vi "TCP.IP Server for Ripple Detection - Experiment 2.vi"() -> ()   [LabVIEW 2021]
doc: "Demonstrates how to set up a basic TCP connection, send data to the specified port once a connection has been established, and terminate the connection once the data has been sent. This VI is designed to stop if the TCP connection is terminated. The data sent in this example is an array of random numbers."
panel:
  in  "Number of row to read \nat a time":i32=10000
  in  "File Path":path
  out "Iteration terminal":i32
  in  "Stop 2":bool
  in  "Client Closed":string="The client VI closed the connection."
  in  "Stop":bool
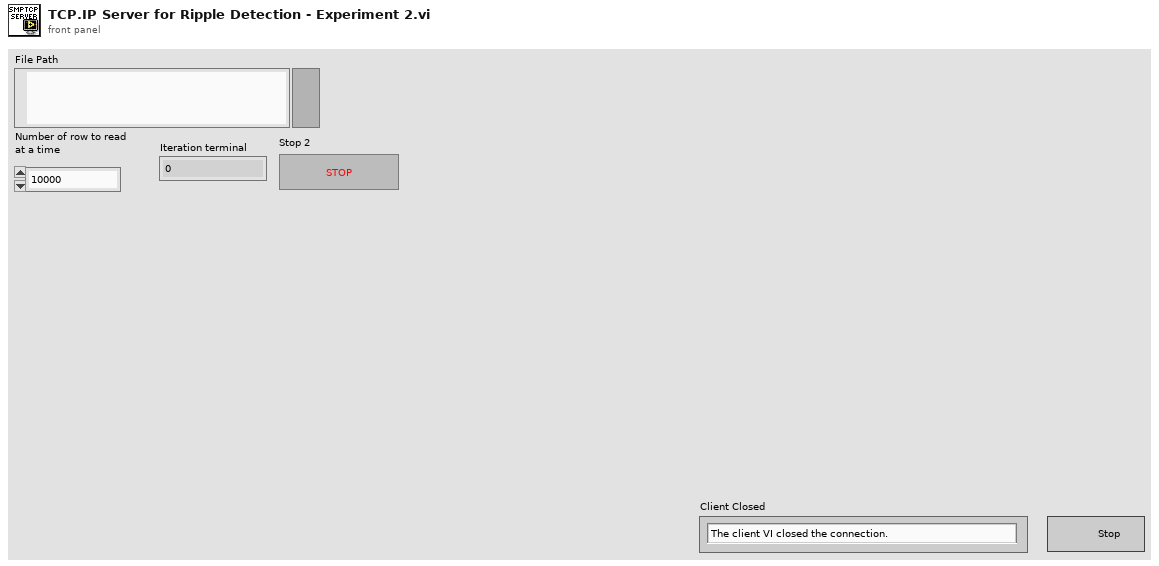
[diagram p1: front panel]
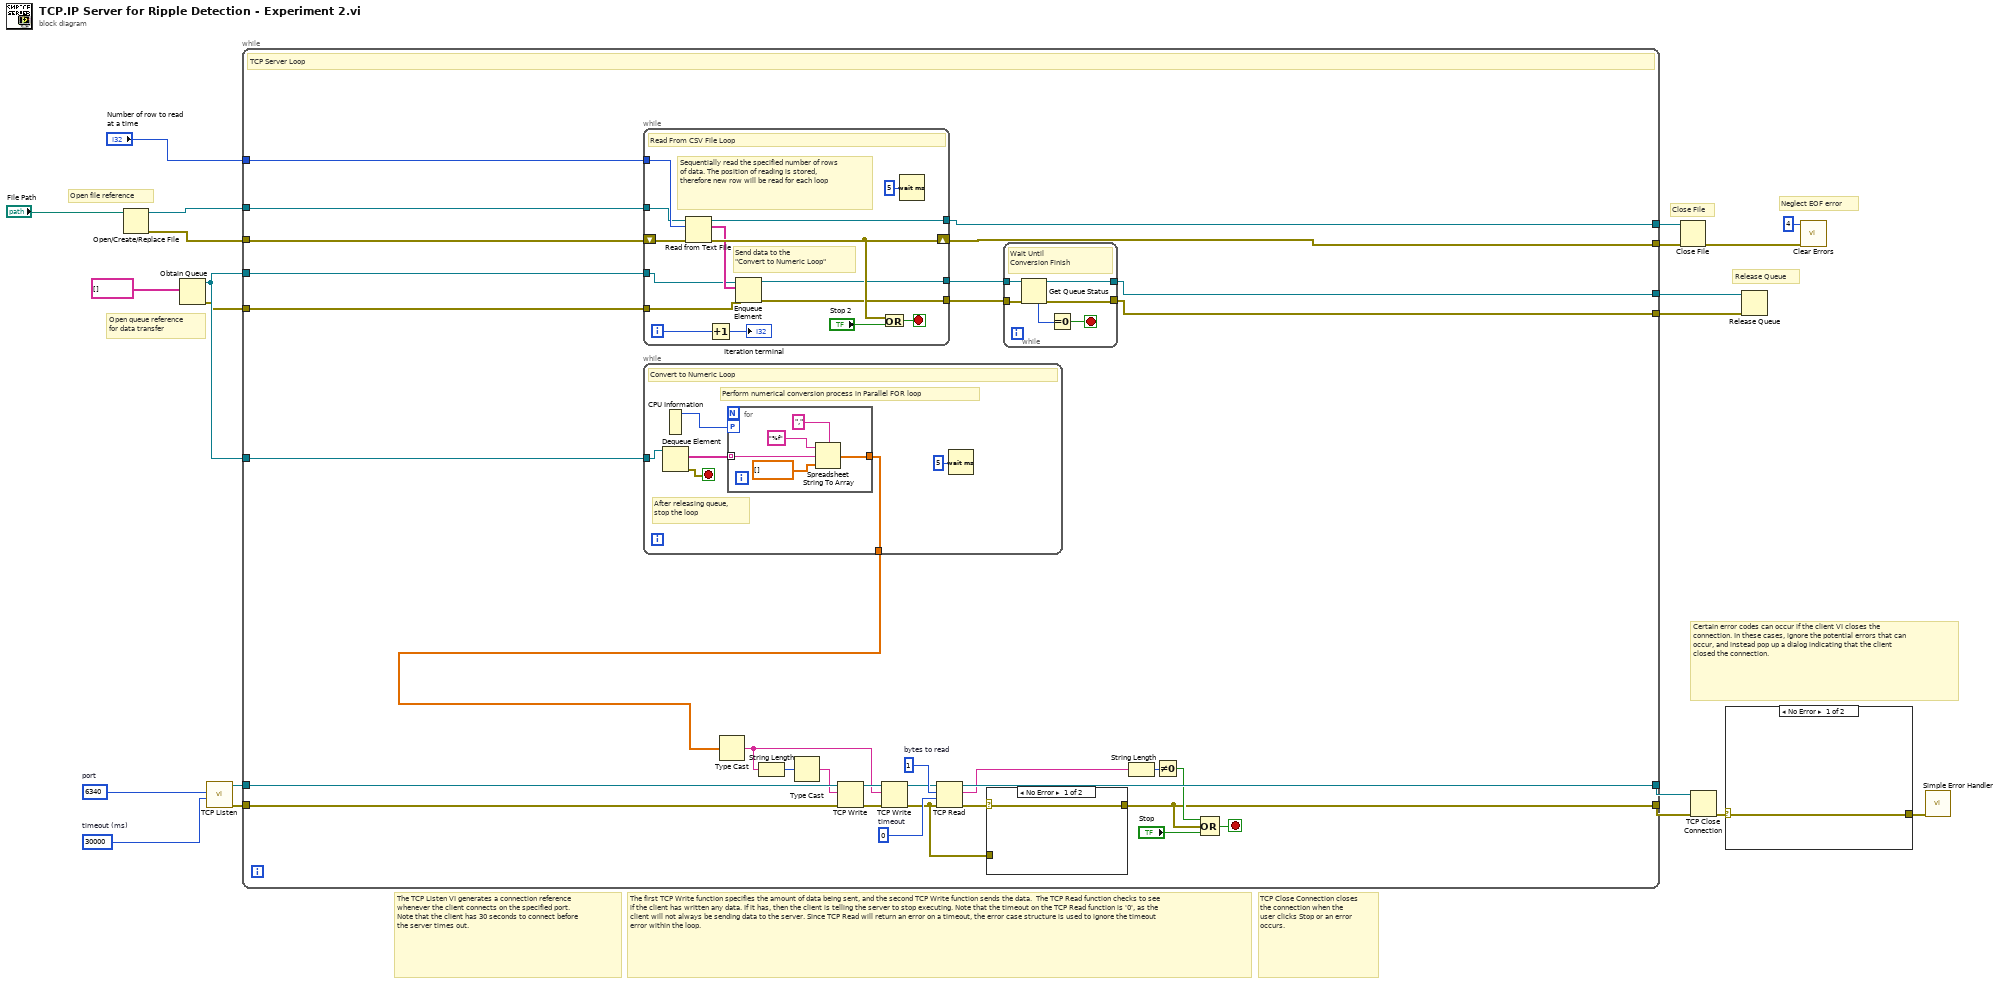
[diagram p0: block diagram]
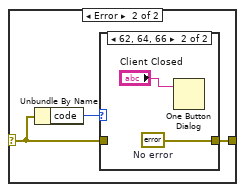
[diagram p2: hidden frame]
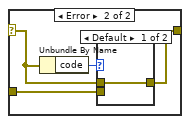
[diagram p4: hidden frame]
diagram:
  w14 = u16 6340  # port
  w15 = 30000  # timeout (ms)
  # "Open queue reference\nfor data transfer"
  # "Release Queue"
  # "Neglect EOF error"
  # "Close File"
  # "Open file reference"
  # "TCP Close Connection closes the connection when the user clicks Stop or an error occurs."
  # "The TCP Listen VI generates a connection reference whenever the client connects on the specified port. Note that the client has 30 seconds to connect before the server times out."
  # "Certain error codes can occur if the client VI closes the connection. In these cases, ignore the potential errors that can occur, and instead pop up a dialog indicating that the client closed the connection."
  # "The first TCP Write function specifies the amount of data being sent, and the second TCP Write function sends the data.  The TCP Read function checks to see if the client has written any data. If it has, then the client is telling the server to stop executing. Note that the timeout on the TCP Read function is '0', as the client will not always be sending data to the server. Since TCP Read will return an error on a timeout, the error case structure is used to ignore the timeout error within the loop."
  n1 = Open/Create/Replace File(file path (use dialog)="File Path") -> (refnum out=w11:refnum<file>, error out=w12:errorcluster)  [unwired: 5 in, 1 out]
  n2 = Obtain Queue(element data type=string[] [] ("形式文字列")) -> (queue out=w3:refnum<queue>, error out=w2:errorcluster)  [unwired: 4 in, 1 out]
  n3 = call <vilib>:"TCP Listen.vi"("timeout ms (wait forever: -1)"=w15, "port"=w14) -> ("error out"=w16:errorcluster, "connection ID"=w17:refnum<k5>)  [unwired: 5 in, 3 out]
  n4 = while {
    tunnel: [w36] -> w20
    tunnel: [w42] -> w21
    tunnel: w17 -> [w53]
    tunnel: w16 -> [w46]
    tunnel: w11 -> [w31]
    tunnel: w12 -> [w30]
    tunnel: [w29] -> w9
    tunnel: [w28] -> w8
    tunnel: [w27] -> w6
    tunnel: [w26] -> w5
    tunnel: w3 -> [w25]
    tunnel: w3 -> [w24]
    tunnel: w2 -> [w23]
    tunnel: "Number of row to read \nat a time" -> [w22]
    stop <- w47 stop-if-true
    w41 = 0  # timeout
    w44 = 1  # bytes to read
    # "TCP Server Loop"
    n5 = while {
      tunnel: [w73] -> w28
      shift-right: [w68] -> w29
      shift-left: w30 -> [w74]
      tunnel: w22 -> [w69]
      tunnel: [w66] -> w33
      tunnel: [w65] -> w34
      tunnel: w31 -> [w62]
      tunnel: w24 -> [w61]
      tunnel: w23 -> [w60]
      i -> [w71]
      stop <- w72 stop-if-true
      # "Send data to the \n\"Convert to Numeric Loop\""
      # "Sequentially read the specified number of rows of data. The position of reading is stored, therefore new row will be read for each loop"
      # "Read From CSV File Loop"
      n6 = Read from Text File(file (use dialog)=w62, count=w69, error in=w74) -> (refnum out=w73:refnum<file>, text=w67:string[], error out=w68:errorcluster)  [unwired: 1 in, 1 out]
      n7 = Increment(x=w71) -> (x+1=→"Iteration terminal":i32)
      n8 = Enqueue Element(queue=w61, element=w67, error in (no error)=w60) -> (queue out=w66:refnum<queue>, error out=w65:errorcluster)  [unwired: 1 in, 1 out]
      n9 = Or(x=w68, y="Stop 2") -> (x .or. y?=w72:bool)
      n10 = Wait (ms)(milliseconds to wait=u32 5) -> ()  [unwired: 1 out]
    }
    n11 = while {
      tunnel: [w77] -> w32
      tunnel: w25 -> [w75]
      stop <- w79 stop-if-true
      # "After releasing queue,\nstop the loop"
      # "Perform numerical conversion process in Parallel FOR loop"
      # "Convert to Numeric Loop"
      n12 = CPU Information() -> (4:w78:i32)  [unwired: 3 out]
      n13 = Dequeue Element(queue=w75) -> (element=w80:string[], error out=w79:errorcluster)  [unwired: 2 in, 2 out]
      n14 = for "Forループ" {
        tunnel: w80 -> [w82] mode=indexing
        tunnel: [w83] -> w77
        workers-P: w78 -> [_]
        n15 = Spreadsheet String To Array(delimiter (Tab)="," ("デリミタ（タブ）"), format string="%f" ("形式文字列"), spreadsheet string=w82, array type (2D Dbl)=dbl[] []) -> (array=w83:dbl[])
      }
      n16 = Wait (ms)(milliseconds to wait=u32 5) -> ()  [unwired: 1 out]
    }
    n17 = Type Cast(x=w32) -> (*(type *) &x=w48:string)  [unwired: 1 out]
    n18 = String Length(string=w48) -> (length=w50:i32)
    n19 = Type Cast(x=w50) -> (*(type *) &x=w49:string)  [unwired: 1 out]
    n20 = TCP Write(connection ID=w53, data in=w49, error in (no error)=w46) -> (connection ID out=w52:refnum<k5>, error out=w51:errorcluster)  [unwired: 2 out]
    n21 = TCP Write(connection ID=w52, data in=w48, error in (no error)=w51) -> (connection ID out=w43:refnum<k5>, error out=w35:errorcluster)  [unwired: 2 out]
    n22 = TCP Read(connection ID=w43, bytes to read=w44, error in (no error)=w35, 9:w41) -> (connection ID out=w42:refnum<k5>, data out=w39:string, error out=w37:errorcluster)  [unwired: 1 out]
    n23 = case shown="No Error" w37 {
      selector: w37 -> [w86 w89]
      tunnel: [w86 w87] -> w36
      tunnel: w35 -> [_ w88]
      frame No Error {
      }
      frame Error {
        n24 = Unbundle By Name(w89) -> ("code"=w90:i32)
        n25 = case shown="Default" w90 {
          tunnel: w89 -> [w91 _]
          tunnel: w88 -> [_ w92]
          tunnel: [w91 w92] -> w87
          frame Default {
          }
          frame 56 {
          }
        }
      }
    }
    n26 = while {
      tunnel: w33 -> [w59]
      tunnel: w34 -> [w58]
      tunnel: [w55] -> w27
      tunnel: [w54] -> w26
      stop <- w56 stop-if-true
      # "Wait Until \nConversion Finish"
      n27 = Get Queue Status(queue=w59, error in (no error)=w58) -> (queue out=w55:refnum<queue>, error out=w54:errorcluster, # elements in queue=w57:i32)  [unwired: 1 in, 5 out]
      n28 = Equal To 0?(x=w57) -> (x = 0?=w56:bool)
    }
    n29 = String Length(string=w39) -> (length=w40:i32)
    n30 = Not Equal To 0?(x=w40) -> (x != 0?=w38:bool)
    n31 = Compound Arithmetic op=OR(w38, w36, "Stop") -> (w47:bool)
  }
  n32 = Close File(refnum=w8, error in=w9) -> (error out=w10:errorcluster)  [unwired: 1 out]
  n33 = TCP Close Connection(connection ID=w21, error in (no error)=w20) -> (error out=w19:errorcluster)  [unwired: 2 out]
  n34 = case shown="No Error" w19 {
    selector: w19 -> [w93 w95]
    tunnel: [w93 w94] -> w18
    frame No Error {
    }
    frame Error {
      n35 = Unbundle By Name(w95) -> ("code"=w96:i32)
      n36 = case shown="62, 64, 66" w96 {
        tunnel: w95 -> [w97 _]
        tunnel: [w97 w99] -> w94
        frame Default {
        }
        frame 62, 64, 66 {
          w99 = errorcluster {"status"=FALSE, "code"=0, "source"=""}  # No error
          n37 = One Button Dialog(message="Client Closed") -> ()  [unwired: 1 in, 1 out]
        }
      }
    }
  }
  n38 = Release Queue(queue=w6, error in (no error)=w5) -> ()  [unwired: 1 in, 3 out]
  n39 = call <vilib>:"Clear Errors.vi"("error in (no error)"=w10, "specific error code to clear (0: all)"=4) -> ()  [unwired: 4 in, 2 out]
  n40 = call <vilib>:"Simple Error Handler.vi"("error in (no error)"=w18) -> ()  [unwired: 1 in, 8 out]
